vi "SP Convert 4.4 - 4.5 to 5.0.vi"(0 "S Parameter 4.4 - 4.5 Test Parameters":T2={"Stimulus"={"Use Instrument Settings"=FALSE, "Blank Frequencies"=FALSE, "Sweep Type"=enum."Linear", "Sweep"={"Fstart"=0.0, "Fstop"=0.0, "Units"=enum."Hz", "Points"=2}, "Power (dBm)"=999.0, "IFBW (Hz)"=-1.0, "Sweep Time (s)"=-1.0}, "Measurement"={"Auto Select"=FALSE, "Data Source"=enum."VNA", "Ports"=2, "Calibration"={"State"=FALSE, "String"=""}, "Parameters"=[]}, "De-Embed"={"De-Embed"=FALSE, "Adapters"=[]}, "Display"={"Lock Control"=FALSE, "Retain Settings"=FALSE, "Formatted Data"=FALSE, "Plot Orientation"=enum."Single", "Plot Controls"=[{"Trace Orientation"=enum."Overlay", "Frequency"={"Change Frequency"=FALSE, "Start"=500.0, "Stop"=1500.0, "Units"=enum."MHz"}, "Markers (MHz)"=[], "Traces"=[{"Trace On"=TRUE, "Measure"=0, "Format"=0, "Autoscale"=TRUE, "Reference"=0.0, "\nRefUnit"="dB/Div", "Position"=5.0, "Scale"=10.0, "ScaleUnit"="dB/Div", "LimitOn"=TRUE, "LimitFill"=FALSE, "Display Data"=0, "Show Markers"=FALSE, "SXX"=""}, {"Trace On"=TRUE, "Measure"=0, "Format"=0, "Autoscale"=TRUE, "Reference"=0.0, "\nRefUnit"="dB/Div", "Position"=5.0, "Scale"=10.0, "ScaleUnit"="dB/Div", "LimitOn"=TRUE, "LimitFill"=FALSE, "Display Data"=0, "Show Markers"=FALSE, "SXX"=""}]}, {"Trace Orientation"=enum."Overlay", "Frequency"={"Change Frequency"=FALSE, "Start"=500.0, "Stop"=1500.0, "Units"=enum."MHz"}, "Markers (MHz)"=[], "Traces"=[{"Trace On"=TRUE, "Measure"=0, "Format"=0, "Autoscale"=TRUE, "Reference"=0.0, "\nRefUnit"="dB/Div", "Position"=5.0, "Scale"=10.0, "ScaleUnit"="dB/Div", "LimitOn"=TRUE, "LimitFill"=FALSE, "Display Data"=0, "Show Markers"=FALSE, "SXX"=""}, {"Trace On"=TRUE, "Measure"=0, "Format"=0, "Autoscale"=TRUE, "Reference"=0.0, "\nRefUnit"="dB/Div", "Position"=5.0, "Scale"=10.0, "ScaleUnit"="dB/Div", "LimitOn"=TRUE, "LimitFill"=FALSE, "Display Data"=0, "Show Markers"=FALSE, "SXX"=""}]}, {"Trace Orientation"=enum."Overlay", "Frequency"={"Change Frequency"=FALSE, "Start"=500.0, "Stop"=1500.0, "Units"=enum."MHz"}, "Markers (MHz)"=[], "Traces"=[{"Trace On"=TRUE, "Measure"=0, "Format"=0, "Autoscale"=TRUE, "Reference"=0.0, "\nRefUnit"="dB/Div", "Position"=5.0, "Scale"=10.0, "ScaleUnit"="dB/Div", "LimitOn"=TRUE, "LimitFill"=FALSE, "Display Data"=0, "Show Markers"=FALSE, "SXX"=""}, {"Trace On"=TRUE, "Measure"=0, "Format"=0, "Autoscale"=TRUE, "Reference"=0.0, "\nRefUnit"="dB/Div", "Position"=5.0, "Scale"=10.0, "ScaleUnit"="dB/Div", "LimitOn"=TRUE, "LimitFill"=FALSE, "Display Data"=0, "Show Markers"=FALSE, "SXX"=""}]}, {"Trace Orientation"=enum."Overlay", "Frequency"={"Change Frequency"=FALSE, "Start"=500.0, "Stop"=1500.0, "Units"=enum."MHz"}, "Markers (MHz)"=[], "Traces"=[{"Trace On"=TRUE, "Measure"=0, "Format"=0, "Autoscale"=TRUE, "Reference"=0.0, "\nRefUnit"="dB/Div", "Position"=5.0, "Scale"=10.0, "ScaleUnit"="dB/Div", "LimitOn"=TRUE, "LimitFill"=FALSE, "Display Data"=0, "Show Markers"=FALSE, "SXX"=""}, {"Trace On"=TRUE, "Measure"=0, "Format"=0, "Autoscale"=TRUE, "Reference"=0.0, "\nRefUnit"="dB/Div", "Position"=5.0, "Scale"=10.0, "ScaleUnit"="dB/Div", "LimitOn"=TRUE, "LimitFill"=FALSE, "Display Data"=0, "Show Markers"=FALSE, "SXX"=""}]}]}, "Limits"=[]} {"Measurement"."Parameters"."Channel" min=0 max=32 step=1; "Measurement"."Parameters"."Parameter"."Stimulus Port" min=1 step=1; "Measurement"."Parameters"."Parameter"."Response Port" min=1 step=1; "Limits"."Parameter"."Stimulus Port" min=1 step=1; "Limits"."Parameter"."Response Port" min=1 step=1; "Stimulus"."Sweep Time (s)" format="%.3g"; "Display"."Plot Controls"."Traces"."Reference" format="%#.2g"; "Display"."Plot Controls"."Traces"."Display Data" items=["Data", "Memory", "Data/Memory"]; "Display"."Plot Controls"."Traces"."Format" items=["Log Mag", "Phase", "Expanded Phase", "Delay", "Smith", "Polar", "Lin Mag", "SWR", "Loss", "Real", "Imaginary"]; "Display"."Plot Controls"."Traces"."Scale" min=0.001 step=1.0 format="%#.2g"; "Display"."Plot Controls"."Traces"."Position" min=0.0 max=10.0; "Display"."Plot Controls"."Frequency"."Stop" format="%.3g"; "Display"."Plot Controls"."Frequency"."Start" format="%.3g"}) -> (2 "S Parameter 5.0 Test Parameters":T1={"Stimulus"={"Use Instrument Settings"=FALSE, "Blank Frequencies"=FALSE, "Sweep Type"=enum."Linear", "Sweep"={"Fstart"=500.0, "Fstop"=1500.0, "Units"=enum."MHz", "Points"=2}, "Power (dBm)"=999.0, "IFBW (Hz)"=-1.0, "Sweep Time (s)"=-1.0, "Calibration"={"State"=FALSE, "String"=""}}, "Measurement"={"Auto Select"=TRUE, "Data Source"=enum."VNA", "Ports"=2, "Parameters"=[]}, "De-Embed"={"De-Embed"=FALSE, "Adapters"=[]}, "Display"={"Lock Control"=FALSE, "Retain Settings"=TRUE, "Formatted Data"=FALSE, "Plot Orientation"=enum."Single", "Plot Controls"=[{"Trace Orientation"=enum."Overlay", "Frequency"={"Change Frequency"=FALSE, "Start"=500.0, "Stop"=1500.0, "Units"=enum."MHz"}, "Markers"=[], "Traces"=[]}, {"Trace Orientation"=enum."Overlay", "Frequency"={"Change Frequency"=FALSE, "Start"=500.0, "Stop"=1500.0, "Units"=enum."MHz"}, "Markers"=[], "Traces"=[]}, {"Trace Orientation"=enum."Overlay", "Frequency"={"Change Frequency"=FALSE, "Start"=500.0, "Stop"=1500.0, "Units"=enum."MHz"}, "Markers"=[], "Traces"=[]}, {"Trace Orientation"=enum."Overlay", "Frequency"={"Change Frequency"=FALSE, "Start"=500.0, "Stop"=1500.0, "Units"=enum."MHz"}, "Markers"=[], "Traces"=[]}]}, "Limits"=[], "Filter Limits"=[]} {"Filter Limits"."Parameter"."Stimulus Port" min=1 step=1; "Filter Limits"."Parameter"."Response Port" min=1 step=1; "Filter Limits"."Passband"."Bandwidth Attn" format="%.3g"; "Filter Limits"."Passband"."Stop/Span" format="%.3g"; "Filter Limits"."Passband"."Start/Center" format="%.3g"; "Measurement"."Parameters"."Channel" min=0 max=32 step=1; "Measurement"."Parameters"."Parameter"."Stimulus Port" min=1 step=1; "Measurement"."Parameters"."Parameter"."Response Port" min=1 step=1; "Limits"."Parameter"."Stimulus Port" min=1 step=1; "Limits"."Parameter"."Response Port" min=1 step=1; "Stimulus"."Sweep Time (s)" format="%.3g"; "Display"."Plot Controls"."Traces"."Reference" format="%#.2g"; "Display"."Plot Controls"."Traces"."Display Data" items=["Data", "Memory", "Data/Memory"]; "Display"."Plot Controls"."Traces"."Format" items=["Log Mag", "Phase", "Expanded Phase", "Delay", "Smith", "Polar", "Lin Mag", "SWR", "Loss", "Real", "Imaginary"]; "Display"."Plot Controls"."Traces"."Scale" min=0.001 step=1.0 format="%#.2g"; "Display"."Plot Controls"."Traces"."Position" min=0.0 max=10.0; "Display"."Plot Controls"."Frequency"."Stop" format="%.3g"; "Display"."Plot Controls"."Frequency"."Start" format="%.3g"})   [LabVIEW 2011]
uses:
  TypeDefs/SP Test Parameters v4.4-4.5.ctl
  TypeDefs/SP Test Parameters v5.0.ctl
  TypeDefs/SP Marker Type.ctl
panel:
  # "Div"
  # "Div"
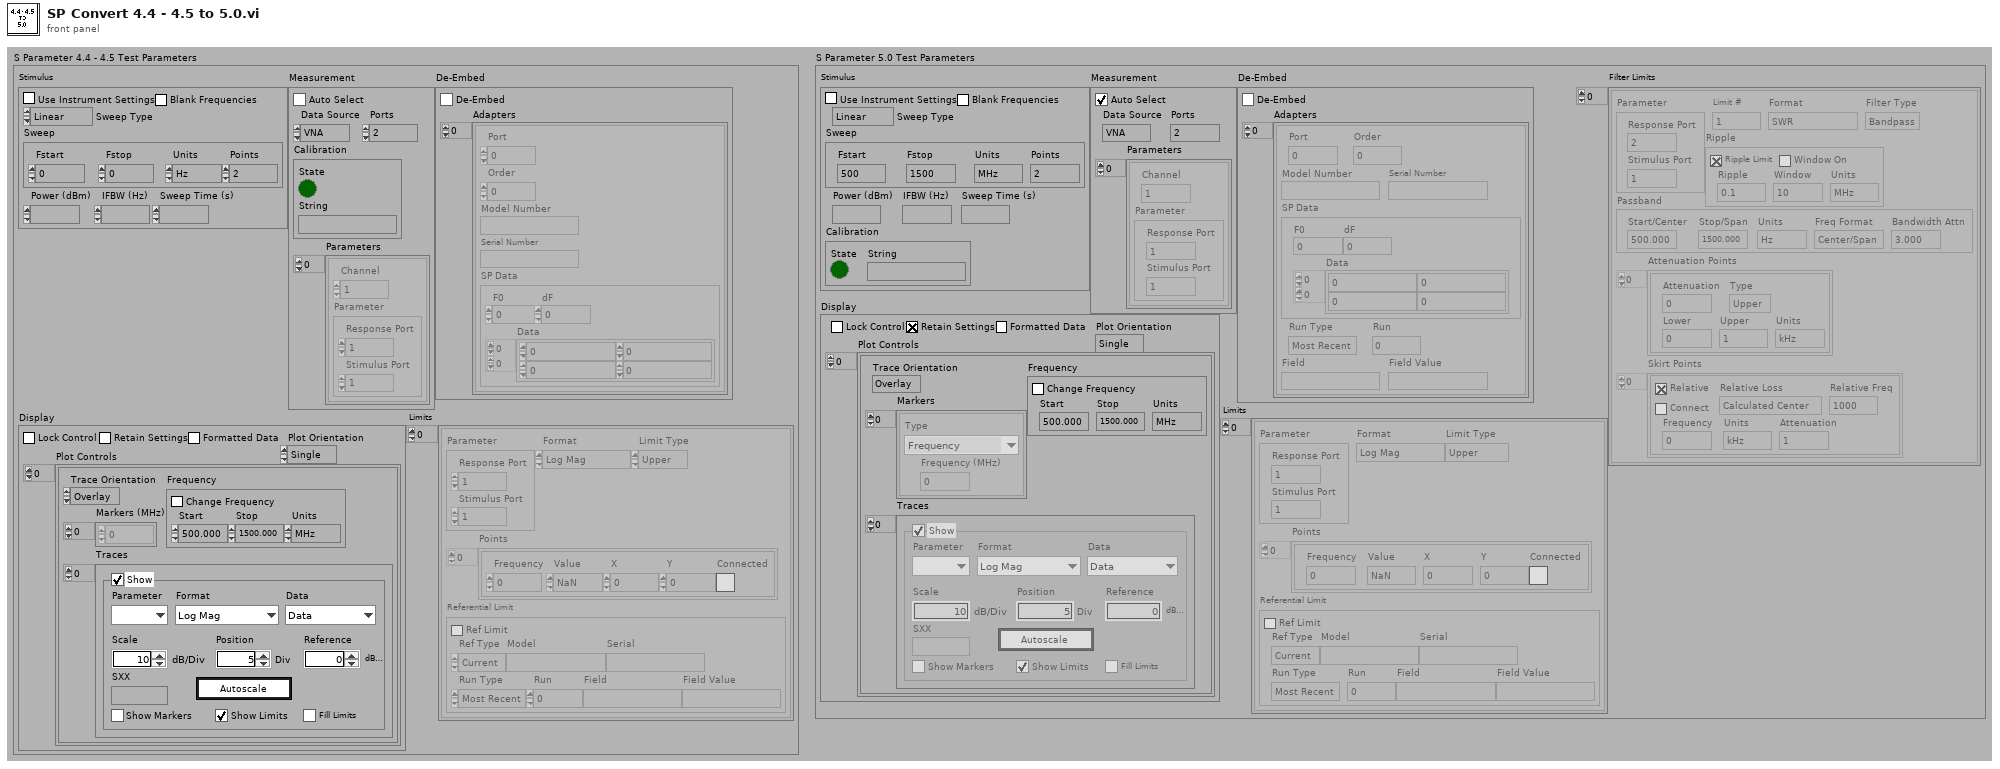
[diagram p1: front panel]
types:
  T1 = typedef "SP Test Parameters v5.0.ctl" = cluster{"Stimulus":cluster{"Use Instrument Settings":bool, "Blank Frequencies":bool, "Sweep Type":enum32{"Linear", "Logarithmic", "List", "Power", "CW"}, "Sweep":cluster{"Fstart":dbl, "Fstop":dbl, "Units":enum16{"Hz", "kHz", "MHz", "GHz", "Points"}, "Points":i32}, "Power (dBm)":dbl, "IFBW (Hz)":dbl, "Sweep Time (s)":dbl, "Calibration":cluster{"State":bool, "String":string}}, "Measurement":cluster{"Auto Select":bool, "Data Source":enum16{"VNA", "Data File"}, "Ports":i8, "Parameters":cluster{"Channel":i8, "Parameter":cluster{"Stimulus Port":i8, "Response Port":i8}}[]}, "De-Embed":cluster{"De-Embed":bool, "Adapters":cluster{"Port":i8, "Order":i8, "Model Number":string, "Serial Number":string, "SP Data":cluster{"F0":dbl, "dF":dbl, "Data":cdb[][]}, "Run Type":enum16{"Most Recent", "Run #", "Match Field"}, "Run":i32, "Field":string, "Field Value":string}[]}, "Display":cluster{"Lock Control":bool, "Retain Settings":bool, "Formatted Data":bool, "Plot Orientation":enum32{"Single", "Dual", "Quad"}, "Plot Controls":cluster{"Trace Orientation":enum32{"Overlay", "Split"}, "Frequency":cluster{"Change Frequency":bool, "Start":dbl, "Stop":dbl, "Units":enum16{"Hz", "kHz", "MHz", "GHz", "Points"}}, "Markers":cluster{"Type":enum16{"Frequency", "Trace Maximum", "Trace Minimum", "Limit Maximum", "Limit Minimum"}, "Frequency (MHz)":dbl}[], "Traces":cluster{"Trace On":bool, "Measure":i32, "Format":i32, "Autoscale":bool, "Reference":dbl, "\nRefUnit":string, "Position":dbl, "Scale":dbl, "ScaleUnit":string, "LimitOn":bool, "LimitFill":bool, "Display Data":u16, "Show Markers":bool, "SXX":string}[]}[]}, "Limits":cluster{"Parameter":cluster{"Stimulus Port":i8, "Response Port":i8}, "Format":enum16{"Log Mag", "Lin Mag", "SWR", "Phase", "Expanded Phase", "Delay", "Insertion Loss", "Isolation", "Return Loss"}, "Limit Type":enum16{"Upper", "Lower", "Delta", "Filter", "Referential"}, "Points":cluster{"Frequency":dbl, "Value":dbl, "X":dbl, "Y":dbl, "Connected":bool}[], "Referential Limit":cluster{"Ref Limit":bool, "Ref Type":enum16{"Current", "Specify"}, "Model":string, "Serial":string, "Run Type":enum16{"Most Recent", "Run #", "Match Field"}, "Run":i32, "Field":string, "Field Value":string}}[], "Filter Limits":cluster{"Limit #":i8, "Parameter":cluster{"Stimulus Port":i8, "Response Port":i8}, "Format":enum16{"Log Mag", "Lin Mag", "SWR", "Phase", "Expanded Phase", "Delay", "Insertion Loss", "Isolation", "Return Loss"}, "Filter Type":enum16{"Lowpass", "Highpass", "Bandpass", "Bandstop"}, "Passband":cluster{"Start/Center":dbl, "Stop/Span":dbl, "Units":enum16{"Hz", "kHz", "MHz", "GHz", "Points"}, "Freq Format":enum16{"Start/Stop", "Center/Span"}, "Bandwidth Attn":dbl}, "Ripple":cluster{"Ripple Limit":bool, "Window On":bool, "Ripple":dbl, "Window":dbl, "Units":enum16{"Hz", "kHz", "MHz", "GHz", "Points"}}, "Attenuation Points":cluster{"Attenuation":dbl, "Type":enum16{"Center", "Lower", "Upper"}, "Lower":dbl, "Upper":dbl, "Units":enum16{"Hz", "kHz", "MHz", "GHz", "Points"}}[], "Skirt Points":cluster{"Relative":bool, "Connect":bool, "Frequency":dbl, "Units":enum16{"Hz", "kHz", "MHz", "GHz", "Points"}, "Attenuation":dbl, "Relative Loss":enum16{"Calculated Center", "Passband Minimum", "Passband Maximum", "Passband Average", "Frequency"}, "Relative Freq":dbl}[]}[]}
  T2 = typedef "SP Test Parameters v4.4-4.5.ctl" = cluster{"Stimulus":cluster{"Use Instrument Settings":bool, "Blank Frequencies":bool, "Sweep Type":enum32{"Linear", "Logarithmic", "List", "Power", "CW"}, "Sweep":cluster{"Fstart":dbl, "Fstop":dbl, "Units":enum16{"Hz", "kHz", "MHz", "GHz", "Points"}, "Points":i32}, "Power (dBm)":dbl, "IFBW (Hz)":dbl, "Sweep Time (s)":dbl}, "Measurement":cluster{"Auto Select":bool, "Data Source":enum16{"VNA", "Data File"}, "Ports":i8, "Calibration":cluster{"State":bool, "String":string}, "Parameters":cluster{"Channel":i8, "Parameter":cluster{"Stimulus Port":i8, "Response Port":i8}}[]}, "De-Embed":cluster{"De-Embed":bool, "Adapters":cluster{"Port":i8, "Order":i8, "Model Number":string, "Serial Number":string, "SP Data":cluster{"F0":dbl, "dF":dbl, "Data":cdb[][]}}[]}, "Display":cluster{"Lock Control":bool, "Retain Settings":bool, "Formatted Data":bool, "Plot Orientation":enum32{"Single", "Dual", "Quad"}, "Plot Controls":cluster{"Trace Orientation":enum32{"Overlay", "Split"}, "Frequency":cluster{"Change Frequency":bool, "Start":dbl, "Stop":dbl, "Units":enum16{"Hz", "kHz", "MHz", "GHz", "Points"}}, "Markers (MHz)":dbl[], "Traces":cluster{"Trace On":bool, "Measure":i32, "Format":i32, "Autoscale":bool, "Reference":dbl, "\nRefUnit":string, "Position":dbl, "Scale":dbl, "ScaleUnit":string, "LimitOn":bool, "LimitFill":bool, "Display Data":u16, "Show Markers":bool, "SXX":string}[]}[]}, "Limits":cluster{"Parameter":cluster{"Stimulus Port":i8, "Response Port":i8}, "Format":enum16{"Log Mag", "Lin Mag", "SWR", "Phase", "Expanded Phase", "Delay", "Insertion Loss", "Isolation", "Return Loss"}, "Limit Type":enum16{"Upper", "Lower", "Delta"}, "Points":cluster{"Frequency":dbl, "Value":dbl, "X":dbl, "Y":dbl, "Connected":bool}[], "Referential Limit":cluster{"Ref Limit":bool, "Ref Type":enum16{"Current", "Specify"}, "Model":string, "Serial":string, "Run Type":enum16{"Most Recent", "Run #", "Match Field"}, "Run":i32, "Field":string, "Field Value":string}}[]}
  T3 = enum32{"Linear", "Logarithmic", "List", "Power", "CW"}
  T4 = cluster{"Fstart":dbl, "Fstop":dbl, "Units":enum16{"Hz", "kHz", "MHz", "GHz", "Points"}, "Points":i32}
  T5 = cluster{"Channel":i8, "Parameter":cluster{"Stimulus Port":i8, "Response Port":i8}}[]
  T6 = cluster{"Parameter":cluster{"Stimulus Port":i8, "Response Port":i8}, "Format":enum16{"Log Mag", "Lin Mag", "SWR", "Phase", "Expanded Phase", "Delay", "Insertion Loss", "Isolation", "Return Loss"}, "Limit Type":enum16{"Upper", "Lower", "Delta"}, "Points":cluster{"Frequency":dbl, "Value":dbl, "X":dbl, "Y":dbl, "Connected":bool}[], "Referential Limit":cluster{"Ref Limit":bool, "Ref Type":enum16{"Current", "Specify"}, "Model":string, "Serial":string, "Run Type":enum16{"Most Recent", "Run #", "Match Field"}, "Run":i32, "Field":string, "Field Value":string}}[]
  T7 = cluster{"Trace Orientation":enum32{"Overlay", "Split"}, "Frequency":cluster{"Change Frequency":bool, "Start":dbl, "Stop":dbl, "Units":enum16{"Hz", "kHz", "MHz", "GHz", "Points"}}, "Markers (MHz)":dbl[], "Traces":cluster{"Trace On":bool, "Measure":i32, "Format":i32, "Autoscale":bool, "Reference":dbl, "\nRefUnit":string, "Position":dbl, "Scale":dbl, "ScaleUnit":string, "LimitOn":bool, "LimitFill":bool, "Display Data":u16, "Show Markers":bool, "SXX":string}[]}[]
  T8 = cluster{"Port":i8, "Order":i8, "Model Number":string, "Serial Number":string, "SP Data":cluster{"F0":dbl, "dF":dbl, "Data":cdb[][]}}[]
  T9 = cluster{"Trace Orientation":enum32{"Overlay", "Split"}, "Frequency":cluster{"Change Frequency":bool, "Start":dbl, "Stop":dbl, "Units":enum16{"Hz", "kHz", "MHz", "GHz", "Points"}}, "Markers":cluster{"Type":enum16{"Frequency", "Trace Maximum", "Trace Minimum", "Limit Maximum", "Limit Minimum"}, "Frequency (MHz)":dbl}[], "Traces":cluster{"Trace On":bool, "Measure":i32, "Format":i32, "Autoscale":bool, "Reference":dbl, "\nRefUnit":string, "Position":dbl, "Scale":dbl, "ScaleUnit":string, "LimitOn":bool, "LimitFill":bool, "Display Data":u16, "Show Markers":bool, "SXX":string}[]}[]
  T10 = cluster{"Port":i8, "Order":i8, "Model Number":string, "Serial Number":string, "SP Data":cluster{"F0":dbl, "dF":dbl, "Data":cdb[][]}, "Run Type":enum16{"Most Recent", "Run #", "Match Field"}, "Run":i32, "Field":string, "Field Value":string}[]
  T11 = cluster{"Trace Orientation":enum32{"Overlay", "Split"}, "Frequency":cluster{"Change Frequency":bool, "Start":dbl, "Stop":dbl, "Units":enum16{"Hz", "kHz", "MHz", "GHz", "Points"}}, "Markers":cluster{"Type":enum16{"Frequency", "Trace Maximum", "Trace Minimum", "Limit Maximum", "Limit Minimum"}, "Frequency (MHz)":dbl}[], "Traces":cluster{"Trace On":bool, "Measure":i32, "Format":i32, "Autoscale":bool, "Reference":dbl, "\nRefUnit":string, "Position":dbl, "Scale":dbl, "ScaleUnit":string, "LimitOn":bool, "LimitFill":bool, "Display Data":u16, "Show Markers":bool, "SXX":string}[]}
  T12 = cluster{"Port":i8, "Order":i8, "Model Number":string, "Serial Number":string, "SP Data":cluster{"F0":dbl, "dF":dbl, "Data":cdb[][]}, "Run Type":enum16{"Most Recent", "Run #", "Match Field"}, "Run":i32, "Field":string, "Field Value":string}
  T13 = typedef "SP Marker Type.ctl" = enum16{"Frequency", "Trace Maximum", "Trace Minimum", "Limit Maximum", "Limit Minimum"}
  T14 = cluster{"Type":enum16{"Frequency", "Trace Maximum", "Trace Minimum", "Limit Maximum", "Limit Minimum"}, "Frequency (MHz)":dbl}[]
  T15 = cluster{"Change Frequency":bool, "Start":dbl, "Stop":dbl, "Units":enum16{"Hz", "kHz", "MHz", "GHz", "Points"}}
  T16 = cluster{"Trace On":bool, "Measure":i32, "Format":i32, "Autoscale":bool, "Reference":dbl, "\nRefUnit":string, "Position":dbl, "Scale":dbl, "ScaleUnit":string, "LimitOn":bool, "LimitFill":bool, "Display Data":u16, "Show Markers":bool, "SXX":string}[]
  T17 = cluster{"Type":enum16{"Frequency", "Trace Maximum", "Trace Minimum", "Limit Maximum", "Limit Minimum"}, "Frequency (MHz)":dbl}
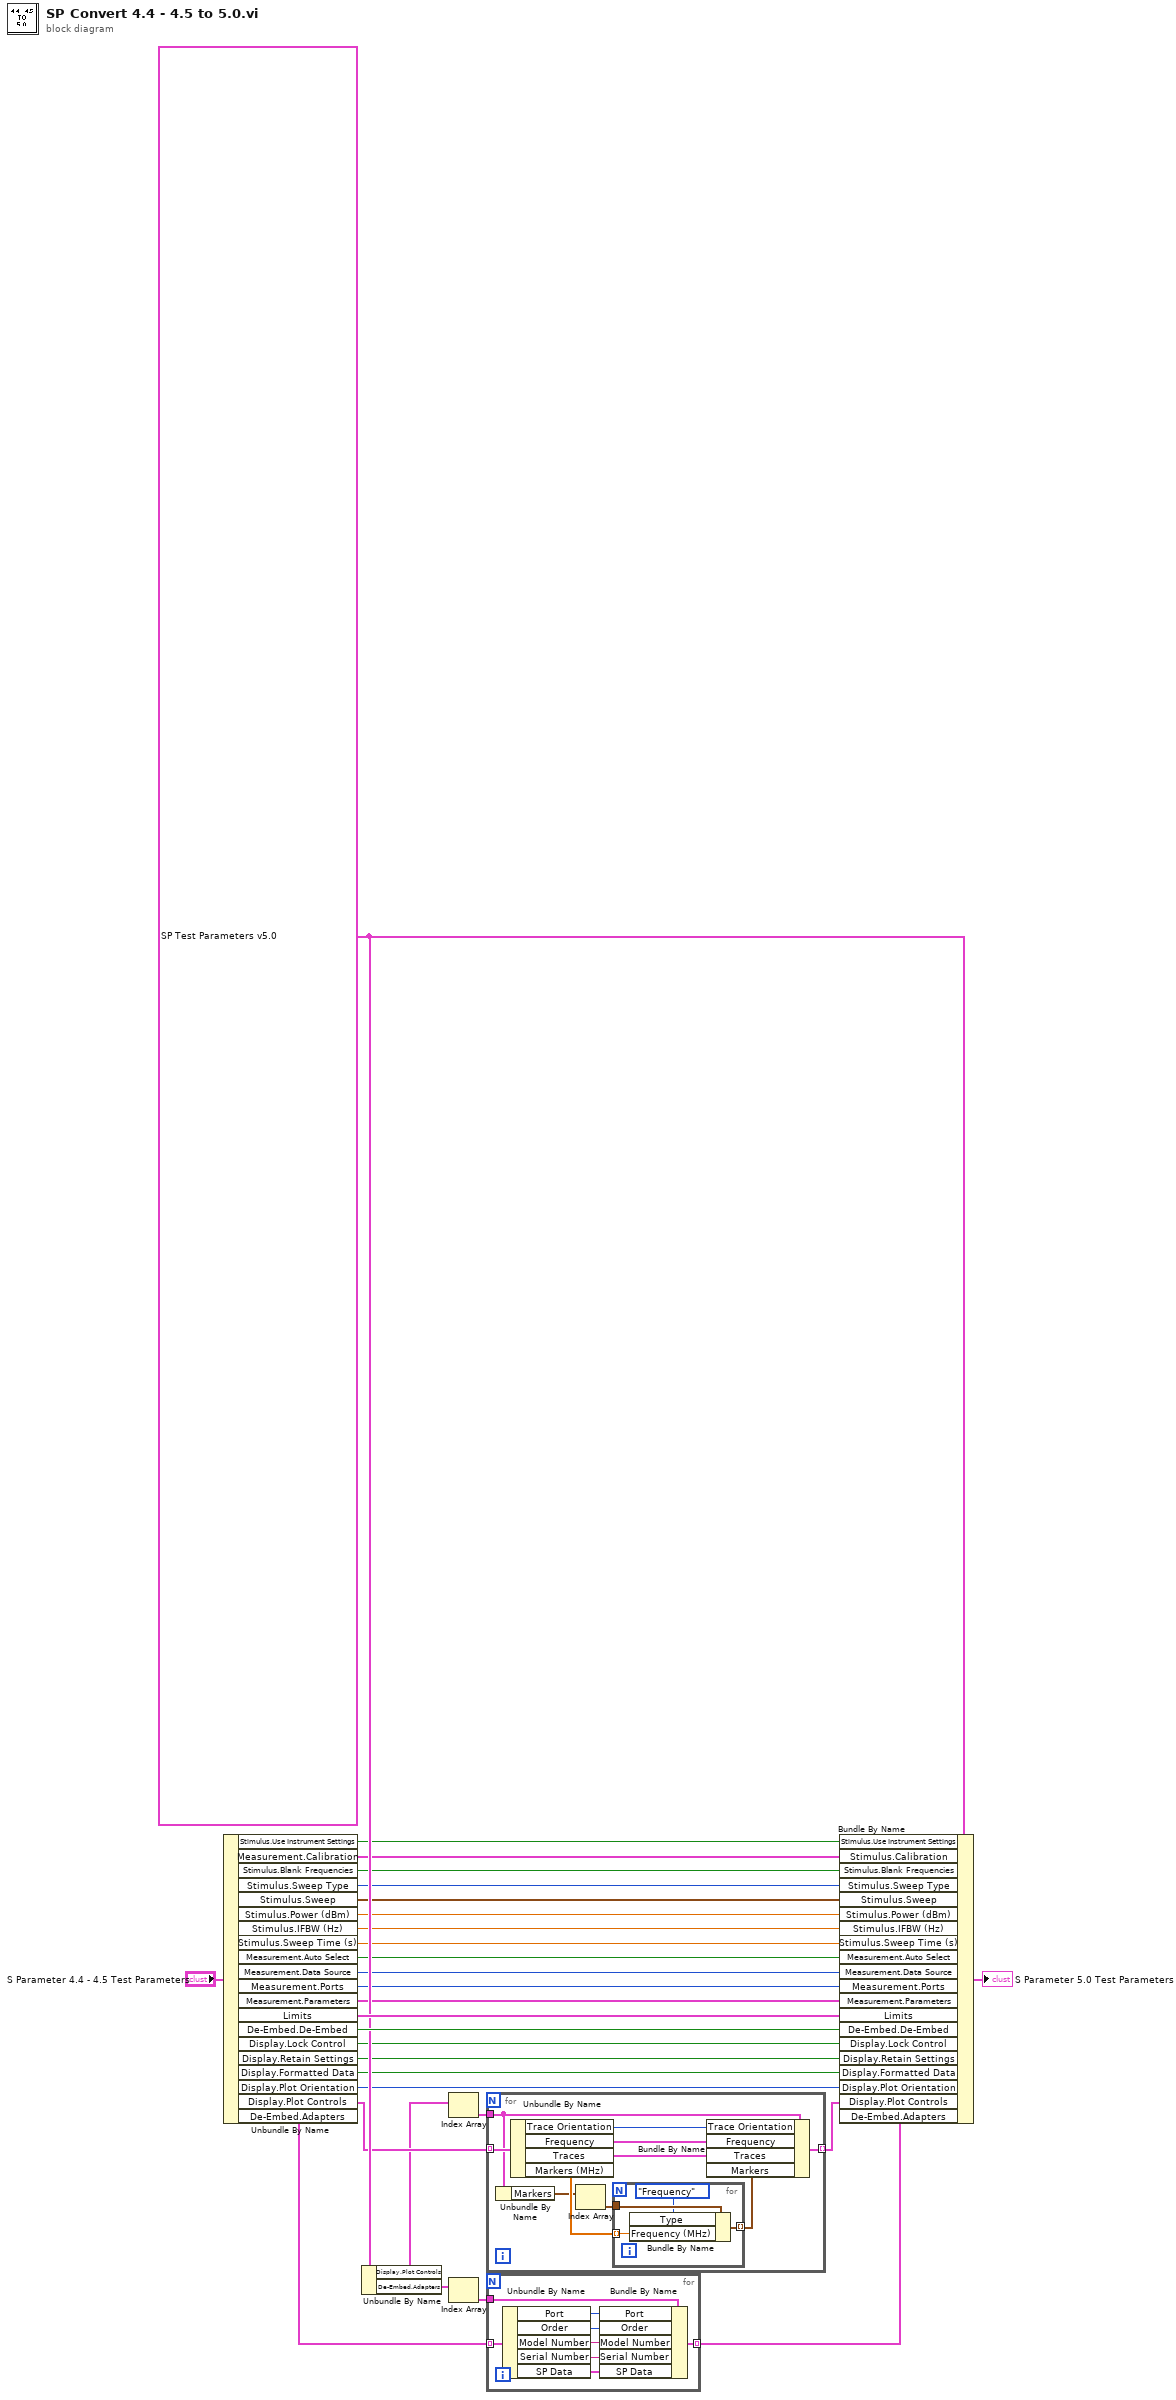
[diagram p0: block diagram]
diagram:
  w25 = T1 {"Stimulus"={"Use Instrument Settings"=FALSE, "Blank Frequencies"=FALSE, "Sweep Type"=enum."Linear", "Sweep"={"Fstart"=0.0, "Fstop"=0.0, "Units"=enum."Hz", "Points"=0}, "Power (dBm)"=0.0, "IFBW (Hz)"=0.0, "Sweep Time (s)"=0.0, "Calibration"={"State"=FALSE, "String"=""}}, "Measurement"={"Auto Select"=FALSE, "Data Source"=enum."VNA", "Ports"=0, "Parameters"=[]}, "De-Embed"={"De-Embed"=FALSE, "Adapters"=[]}, "Display"={"Lock Control"=FALSE, "Retain Settings"=FALSE, "Formatted Data"=FALSE, "Plot Orientation"=enum."Single", "Plot Controls"=[{"Trace Orientation"=enum."Overlay", "Frequency"={"Change Frequency"=FALSE, "Start"=0.0, "Stop"=0.0, "Units"=enum."Hz"}, "Markers"=[], "Traces"=[{"Trace On"=TRUE, "Measure"=0, "Format"=0, "Autoscale"=TRUE, "Reference"=0.0, "\nRefUnit"="dB/Div", "Position"=5.0, "Scale"=10.0, "ScaleUnit"="dB/Div", "LimitOn"=TRUE, "LimitFill"=FALSE, "Display Data"=0, "Show Markers"=FALSE, "SXX"="S11"}, {"Trace On"=TRUE, "Measure"=0, "Format"=0, "Autoscale"=TRUE, "Reference"=0.0, "\nRefUnit"="dB/Div", "Position"=5.0, "Scale"=10.0, "ScaleUnit"="dB/Div", "LimitOn"=TRUE, "LimitFill"=FALSE, "Display Data"=0, "Show Markers"=FALSE, "SXX"="S21"}]}, {"Trace Orientation"=enum."Overlay", "Frequency"={"Change Frequency"=FALSE, "Start"=0.0, "Stop"=0.0, "Units"=enum."Hz"}, "Markers"=[], "Traces"=[{"Trace On"=TRUE, "Measure"=0, "Format"=0, "Autoscale"=TRUE, "Reference"=0.0, "\nRefUnit"="dB/Div", "Position"=5.0, "Scale"=10.0, "ScaleUnit"="dB/Div", "LimitOn"=TRUE, "LimitFill"=FALSE, "Display Data"=0, "Show Markers"=FALSE, "SXX"="S11"}, {"Trace On"=TRUE, "Measure"=0, "Format"=0, "Autoscale"=TRUE, "Reference"=0.0, "\nRefUnit"="dB/Div", "Position"=5.0, "Scale"=10.0, "ScaleUnit"="dB/Div", "LimitOn"=TRUE, "LimitFill"=FALSE, "Display Data"=0, "Show Markers"=FALSE, "SXX"="S21"}]}, {"Trace Orientation"=enum."Overlay", "Frequency"={"Change Frequency"=FALSE, "Start"=0.0, "Stop"=0.0, "Units"=enum."Hz"}, "Markers"=[], "Traces"=[{"Trace On"=TRUE, "Measure"=0, "Format"=0, "Autoscale"=TRUE, "Reference"=0.0, "\nRefUnit"="dB/Div", "Position"=5.0, "Scale"=10.0, "ScaleUnit"="dB/Div", "LimitOn"=TRUE, "LimitFill"=FALSE, "Display Data"=0, "Show Markers"=FALSE, "SXX"="S11"}, {"Trace On"=TRUE, "Measure"=0, "Format"=0, "Autoscale"=TRUE, "Reference"=0.0, "\nRefUnit"="dB/Div", "Position"=5.0, "Scale"=10.0, "ScaleUnit"="dB/Div", "LimitOn"=TRUE, "LimitFill"=FALSE, "Display Data"=0, "Show Markers"=FALSE, "SXX"="S21"}]}, {"Trace Orientation"=enum."Overlay", "Frequency"={"Change Frequency"=FALSE, "Start"=0.0, "Stop"=0.0, "Units"=enum."Hz"}, "Markers"=[], "Traces"=[{"Trace On"=TRUE, "Measure"=0, "Format"=0, "Autoscale"=TRUE, "Reference"=0.0, "\nRefUnit"="dB/Div", "Position"=5.0, "Scale"=10.0, "ScaleUnit"="dB/Div", "LimitOn"=TRUE, "LimitFill"=FALSE, "Display Data"=0, "Show Markers"=FALSE, "SXX"="S11"}, {"Trace On"=TRUE, "Measure"=0, "Format"=0, "Autoscale"=TRUE, "Reference"=0.0, "\nRefUnit"="dB/Div", "Position"=5.0, "Scale"=10.0, "ScaleUnit"="dB/Div", "LimitOn"=TRUE, "LimitFill"=FALSE, "Display Data"=0, "Show Markers"=FALSE, "SXX"="S21"}]}]}, "Limits"=[], "Filter Limits"=[]} ("S Parameter Test Parameters")
  n1 = Unbundle By Name("S Parameter 4.4 - 4.5 Test Parameters") -> ("Stimulus.Use Instrument Settings"=w12:bool, "Measurement.Calibration"=w1:cluster{"State":bool, "String":string}, "Stimulus.Blank Frequencies"=w2:bool, "Stimulus.Sweep Type"=w3:T3, "Stimulus.Sweep"=w4:T4, "Stimulus.Power (dBm)"=w5:dbl, "Stimulus.IFBW (Hz)"=w6:dbl, "Stimulus.Sweep Time (s)"=w7:dbl, "Measurement.Auto Select"=w8:bool, "Measurement.Data Source"=w9:enum16{"VNA", "Data File"}, "Measurement.Ports"=w10:i8, "Measurement.Parameters"=w11:T5, "Limits"=w27:T6, "De-Embed.De-Embed"=w26:bool, "Display.Lock Control"=w20:bool, "Display.Retain Settings"=w19:bool, "Display.Formatted Data"=w18:bool, "Display.Plot Orientation"=w17:enum32{"Single", "Dual", "Quad"}, "Display.Plot Controls"=w16:T7, "De-Embed.Adapters"=w22:T8)
  n2 = Unbundle By Name(w25) -> ("Display.Plot Controls"=w15:T9, "De-Embed.Adapters"=w24:T10)
  n3 = Index Array(array=w15) -> (element=w14:T11)  [unwired: 1 in]
  n4 = Index Array(array=w24) -> (element=w23:T12)  [unwired: 1 in]
  n5 = for {
    tunnel: w16 -> [w39] mode=indexing
    tunnel: w14 -> [w33]
    tunnel: [w38] -> w13 mode=indexing
    n6 = Unbundle By Name(w33) -> ("Markers"=w32:T14)
    n7 = Unbundle By Name(w39) -> ("Trace Orientation"=w37:enum32{"Overlay", "Split"}, "Frequency"=w36:T15, "Traces"=w35:T16, "Markers (MHz)"=w34:dbl[])
    n8 = Index Array(array=w32) -> (element=w31:T17)  [unwired: 1 in]
    n9 = for {
      tunnel: w34 -> [w42] mode=indexing
      tunnel: w31 -> [w43]
      tunnel: [w40] -> w30 mode=indexing
      n10 = Bundle By Name(cluster=w43, "Type"=SP_Marker_Type."Frequency", "Frequency (MHz)"=w42) -> (w40:T17)
    }
    n11 = Bundle By Name(cluster=w33, "Trace Orientation"=w37, "Frequency"=w36, "Traces"=w35, "Markers"=w30) -> (w38:T11)
  }
  n12 = for {
    tunnel: w22 -> [w51] mode=indexing
    tunnel: w23 -> [w50]
    tunnel: [w44] -> w21 mode=indexing
    n13 = Unbundle By Name(w51) -> ("Port"=w49:i8, "Order"=w48:i8, "Model Number"=w47:string, "Serial Number"=w46:string, "SP Data"=w45:cluster{"F0":dbl, "dF":dbl, "Data":cdb[][]})
    n14 = Bundle By Name(cluster=w50, "Port"=w49, "Order"=w48, "Model Number"=w47, "Serial Number"=w46, "SP Data"=w45) -> (w44:T12)
  }
  n15 = Bundle By Name(cluster=w25, "Stimulus.Use Instrument Settings"=w12, "Stimulus.Calibration"=w1, "Stimulus.Blank Frequencies"=w2, "Stimulus.Sweep Type"=w3, "Stimulus.Sweep"=w4, "Stimulus.Power (dBm)"=w5, "Stimulus.IFBW (Hz)"=w6, "Stimulus.Sweep Time (s)"=w7, "Measurement.Auto Select"=w8, "Measurement.Data Source"=w9, "Measurement.Ports"=w10, "Measurement.Parameters"=w11, "Limits"=w27, "De-Embed.De-Embed"=w26, "Display.Lock Control"=w20, "Display.Retain Settings"=w19, "Display.Formatted Data"=w18, "Display.Plot Orientation"=w17, "Display.Plot Controls"=w13, "De-Embed.Adapters"=w21) -> (→"S Parameter 5.0 Test Parameters":T1)
